vi "Get Calibration Deviations.vi"(0 "VISA Session In":refnum<visa-resource-name>="OXYMAT", 1 "Target Address":u8=16 format="%.0x", 2 "Source Address":u8=208 format="%.0x", 11 "error in (no error)":errorcluster) -> (4 "VISA Session Out":refnum<visa-resource-name>, 6 "Message Header":T3 {"Source Address" format="%.0x"; "Target Address" format="%.0x"}, 10 "Deviation":T2={"Zero"={"Measured value"=nan, "Dimension"=enum."Unknown (0)"}, "Slope"={"Measured value"=nan, "Dimension"=enum."Unknown (0)"}} {"Zero"."Measured value" format="%#_6f"; "Slope"."Measured value" format="%#_6f"}, 13 "Success":bool, 15 "error out":errorcluster)   [LabVIEW 2019, in "Siemens ELAN.lvlib"]
doc: "Using the Siemens ELAN protocol, gets calibration deviations from the most recent calibration action. Returns cluster containing measured real values and units of measure for both zero and slope. Also returns a boolean indicating that the addressed device provided a valid response.\n\n$Revision:: 0 $\n$Modtime:: yy-mm-dd hh:mm $\n$Author:: Dboyd $"
uses:
  Siemens ELAN.lvlib
  Unit Dimensions.ctl
  Message Header.ctl
  Channel Status.ctl
panel:
  in  "Dimension":T1
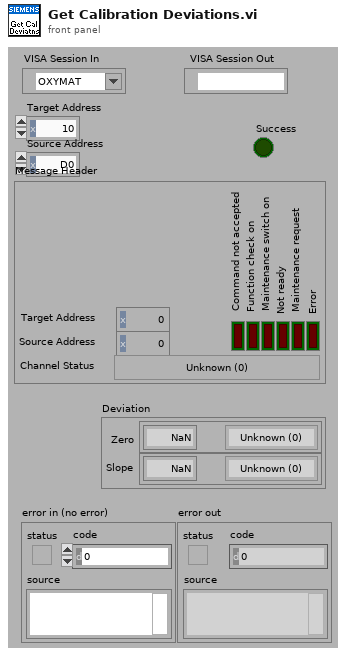
[diagram p1: front panel]
types:
  T1 = typedef "Siemens ELAN.lvlib/Unit Dimensions.ctl" = enum8{"Unknown (0)", "Pure number", "ppm", "ppb", "vpm", "vpm C1", "vpm C3", "vpm C6", "mg C/m^3", "mg/m^3", "%", "% v/v", "% of range", "% saturation", "%/°C", "%/K", "% w/w", "mV/pH", "mV/mbar", "nA/mbar", "S/m", "S/cm", "mS/m", "mS/cm", "uS/m", "uS/cm", "s", "min", "hr", "pA", "mA", "uV", "mV", "V", "mbar", "hPa", "ml/min", "kohm", "MOhm", "S", "°C", "Hz", "pH", "ug/l", "mg/l", "l/min", "uA", "mg/dm^3", "kPa", "kohm*cm", "MOhm*cm", "°", "Unknown (>51)"}
  T2 = cluster{"Zero":cluster{"Measured value":dbl, "Dimension":T1}, "Slope":cluster{"Measured value":dbl, "Dimension":T1}}
  T3 = typedef "Siemens ELAN.lvlib/Message Header.ctl" = cluster{"Target Address":u8, "Source Address":u8, "Error":bool, "Maintenance request":bool, "Not ready":bool, "Maintenance switch on":bool, "Function check on":bool, "Command not accepted":bool, "Channel Status":T4}
  T4 = typedef "Siemens ELAN.lvlib/Channel Status.ctl" = enum8{"Unknown (0)", "Warm-up", "Pause", "Standby", "Measure", "Zero calibration", "Adjust component slope", "Unknown (7)", "Adjust curve dip", "Adjust linearization sensitivity", "Adjust temperature compensation", "Adjust pressure compensation", "Adjust linearization zero", "Adjust flow sensor", "Autocal", "Adjust phase", "Zero calibration of O2 sensor", "Synchronous zero calibration", "Purging for synchronous zero calibration", "Adjust analog output", "Adjust analog input", "Cleaning", "Unknown (>21)"}
  T5 = cluster{"[0]":cluster{"Measured value":dbl, "Dimension":T1}, "[1]":cluster{"Measured value":dbl, "Dimension":T1}}
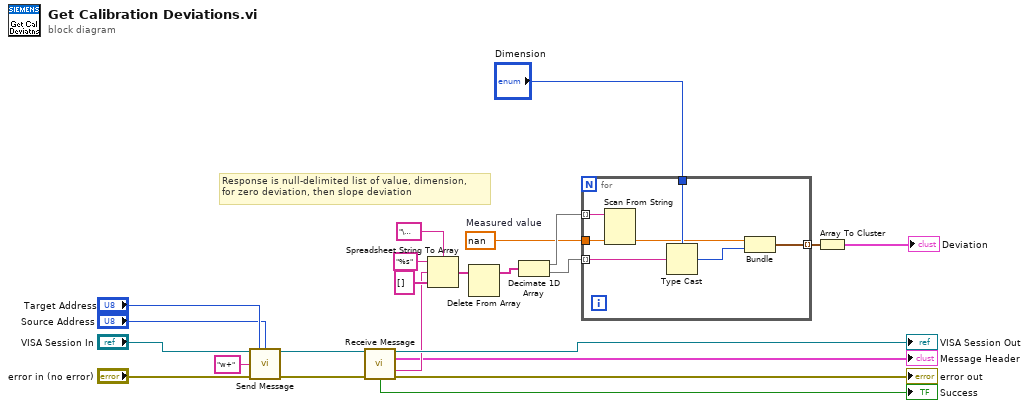
[diagram p0: block diagram]
diagram:
  w5 = nan  # Measured value
  # "Response is null-delimited list of value, dimension,\nfor zero deviation, then slope deviation"
  n1 = call "Send Message.vi"("VISA Session In"="VISA Session In", "Target Address"="Target Address", "Source Address"="Source Address", "Command"="w+", "error in (no error)"="error in (no error)") -> ("VISA Session Out"=w23:refnum<visa-resource-name>, "error out"=w22:errorcluster)  [unwired: 8 in, 1 out]
  n2 = call "Receive Message.vi"("VISA Session In"=w23, "error in (no error)"=w22) -> ("VISA Session Out"=→"VISA Session Out":refnum<visa-resource-name>, "Message Header"=→"Message Header":T3, "Response"=w13:string, "Success"=→"Success":bool, "error out"=→"error out":errorcluster)  [unwired: 8 in, 1 out]
  n3 = Spreadsheet String To Array(delimiter (Tab)="\u0000", format string="%s", spreadsheet string=w13, array type (2D Dbl)=string[] []) -> (array=w10:string[])
  n4 = Delete From Array(array=w10) -> (array with subset deleted=w9:string[])  [unwired: 2 in, 1 out]
  n5 = Decimate 1D Array(w9) -> (w6:string[], w8:string[])
  n6 = for {
    tunnel: "Dimension" -> [w30]
    tunnel: w8 -> [w27] mode=indexing
    tunnel: w6 -> [w29] mode=indexing
    tunnel: w5 -> [w28]
    tunnel: [w24] -> w1 mode=indexing
    n7 = Scan From String(input string=w29, default 1=w28) -> (output 1=w26:dbl)  [unwired: 3 in, 3 out]
    n8 = Type Cast(type=w30, x=w27) -> (*(type *) &x=w25:T1)
    n9 = Bundle("Measured value"=w26, "Dimension"=w25) -> (w24:cluster{"Measured value":dbl, "Dimension":T1})  [unwired: 1 in]
  }
  n10 = Array To Cluster(array=w1) -> (cluster=→"Deviation":T5)
